vi "Update Waveform Segments.vi"(8 "error in (no error)":errorcluster, 11 "Waveform Buffer in":refnum<class "Waveform Buffer.lvclass">) -> (0 "error out":errorcluster, 3 "Waveform Buffer out":refnum<class "Waveform Buffer.lvclass">)   [LabVIEW 2012, in "Waveform Data Logger Engine.lvlib" / "Waveform Buffer.lvclass"]
uses:
  Waveform Buffer.lvclass
  Waveform Buffer.lvclass/Waveform Buffer.ctl
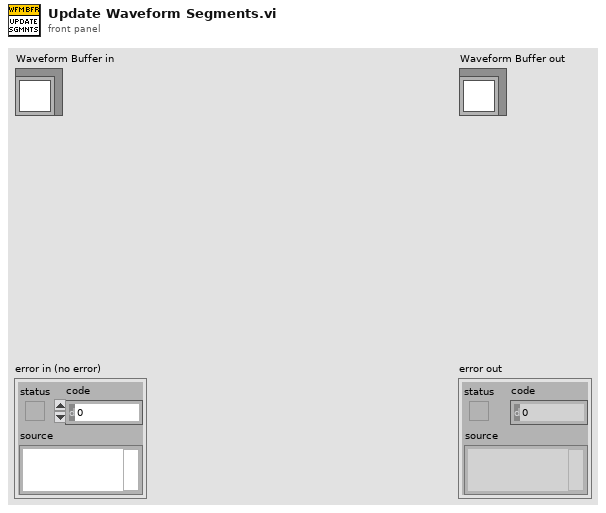
[diagram p1: front panel]
types:
  T1 = typedef "Waveform Data Logger Engine.lvlib/Waveform Buffer.lvclass/Wfm Segment.ctl" = cluster{"ID":u64, "Total samples":i32, "Start":T2, "Finish":T2}
  T2 = typedef "Waveform Data Logger Engine.lvlib/Waveform Buffer.lvclass/Data Point.ctl" = cluster{"Index":i32, "Wfm time":timestamp, "Receive time":timestamp}
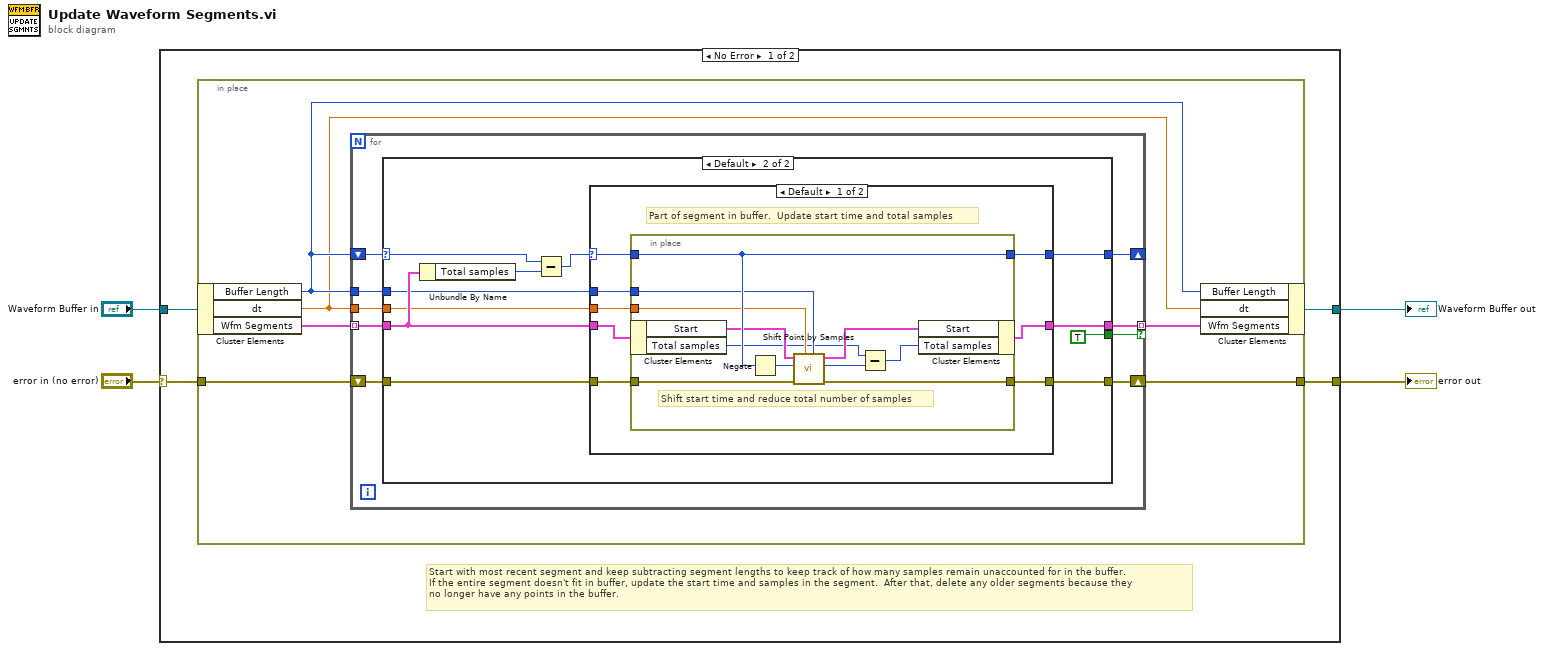
[diagram p0: block diagram]
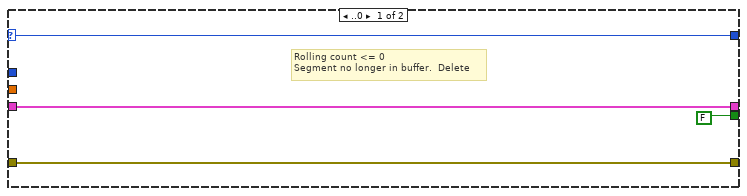
[diagram p2: hidden frame]
diagram:
  n1 = case shown="No Error" "error in (no error)" {
    selector: "error in (no error)" -> [w6 w61]
    tunnel: [w5 w61] -> w1
    tunnel: [w7 w62] -> w2
    tunnel: "Waveform Buffer in" -> [w8 w62]
    frame No Error {
      # "Start with most recent segment and keep subtracting segment lengths to keep track of how many samples remain unaccounted for in the buffer.\nIf the entire segment doesn't fit in buffer, update the start time and samples in the segment.  After that, delete any older segments because they\nno longer have any points in the buffer."
      n2 = in-place {
        in-place-border: w6 -> [w10]
        in-place-border: [w9] -> w5
        n3 = in-place-cluster #1(w8) -> ("Buffer Length"=w13:i32, "dt"=w12:dbl, "Wfm Segments"=w14:T1[])
        n4 = for {
          tunnel: w14 -> [w23] mode=indexing
          tunnel: [w21] -> w11 mode=indexing if=w22
          shift-right: [w20] -> _
          shift-left: w13 -> [w17]
          tunnel: w13 -> [w19]
          tunnel: w12 -> [w18]
          shift-right: [w15] -> w9
          shift-left: w10 -> [w16]
          n5 = case shown="Default" w17 {
            selector: w17 -> [w25 w31]
            tunnel: w23 -> [w27 w35]
            tunnel: [FALSE TRUE] -> w22
            tunnel: [w27 w36] -> w21
            tunnel: [w25 w37] -> w20
            tunnel: w19 -> [_ w34]
            tunnel: w18 -> [_ w33]
            tunnel: w16 -> [w24 w29]
            tunnel: [w24 w28] -> w15
            frame ..0 {
              # "Rolling count <= 0\nSegment no longer in buffer.  Delete"
            }
            frame Default {
              n6 = Unbundle By Name(w35) -> ("Total samples"=w38:i32)
              n7 = Subtract(x=w31, y=w38) -> (x-y=w30:i32)
              n8 = case shown="Default" w30 {
                selector: w30 -> [w41 w59]
                tunnel: [w43 w59] -> w37
                tunnel: [w44 w60] -> w36
                tunnel: w35 -> [w46 w60]
                tunnel: w34 -> [w45 _]
                tunnel: w33 -> [w42 _]
                tunnel: w29 -> [w40 w58]
                tunnel: [w39 w58] -> w28
                frame Default {
                  # "Part of segment in buffer.  Update start time and total samples"
                  n9 = in-place {
                    in-place-border: w41 -> [w57]
                    in-place-border: w42 -> [w53]
                    in-place-border: w45 -> [w52]
                    in-place-border: [w57] -> w43
                    in-place-border: w40 -> [w51]
                    in-place-border: [w50] -> w39
                    # "Shift start time and reduce total number of samples"
                    n10 = in-place-cluster #2(w46) -> ("Start"=w56:T2, "Total samples"=w49:i32)
                    n11 = Negate(x=w57) -> (-x=w54:i32)
                    n12 = call "Shift Point by Samples.vi"("Buffer Length"=w52, "dt"=w53, "error in (no error)"=w51, "Samples"=w54, "Data Point in"=w56) -> ("error out"=w50:errorcluster, "Samples dup"=w47:i32, "Data Point out"=w55:T2)  [unwired: 4 in]
                    n13 = Subtract(x=w49, y=w47) -> (x-y=w48:i32)
                    n14 = in-place-cluster #2("Start"=w55, "Total samples"=w48) -> (w44:T1)
                  }
                }
                frame 0.. {
                  # "Rolling count >= 0\nEntire segment still in buffer"
                }
              }
            }
          }
        }
        n15 = in-place-cluster #1("Buffer Length"=w13, "dt"=w12, "Wfm Segments"=w11) -> (w7:refnum<class "Waveform Buffer.lvclass">)
      }
    }
    frame Error {
    }
  }
  "error out" <- w1
  "Waveform Buffer out" <- w2
